vi "Refresh Targets.vi"(8 "Error In":errorcluster, 11 "Dependency Source Plugins":refnum<class "Dependency Source.lvclass">[](array[class])) -> (0 "Error Out":errorcluster, 1 "All Success?":bool, 2 "Success? Array":bool[](array[boolean]))   [LabVIEW 2019, in "Project.Dependencies Finder.lvlib"]
doc: "Refresh target lists for the given Dependency Source Plugins.\nProvider a Tracker to have a live view of the progress.\n\n2020-12-07: Henrik Dueholm Hansen"
uses:
  Project.Dependencies Finder.lvlib
  Dependency Source/Dependency Source.lvclass
panel:
  out "Target Refresh Progress":i32(slide) scale=0.0..100.0
  # "Refreshing targets. This may take a while.\nClose window to abort"
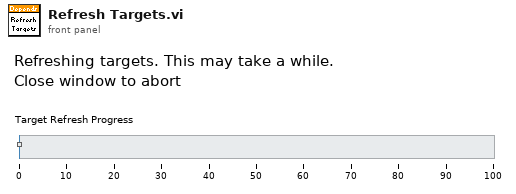
[diagram p1: front panel]
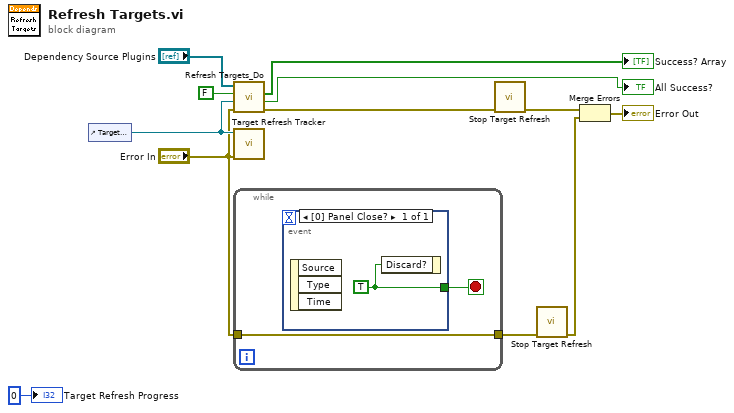
[diagram p0: block diagram]
diagram:
  n1 = control-ref of="Target Refresh Progress"() -> (w7:refnum<vi>)
  n2 = call "Refresh Targets_Do.vi"("Error In"="Error In", "Tracking Progress bar"=w7, "Allow UI?(T)"=FALSE ("Allow UI?"), "Dependency Source Plugins"="Dependency Source Plugins") -> ("Error Out"=w6:errorcluster, "All Success?"=→"All Success?":bool, "Success? Array"=→"Success? Array":bool[])  [unwired: 5 in]
  n3 = call "Target Refresh Tracker.vi"("Error In"="Error In", "Progress bar (auto closed)"=w7) -> ()  [unwired: 10 in]
  n4 = while {
    tunnel: "Error In" -> [w13]
    tunnel: [w13] -> w3
    stop <- w14 stop-if-true
    n5 = event shown="[0] Panel Close?" {
      selector: _ -> [_]
      dyn-events: _ -> [_]
      timeout: _ -> [_]
      tunnel: [w15] -> w14
      event Panel Close? {
        w15 = TRUE
        n6 = event-data() -> ()  [unwired: 1 in, 3 out]
        n7 = event-data("Discard?"=w15) -> ()  [unwired: 1 in, 1 out]
      }
    }
  }
  n8 = call "Stop Target Refresh.vi"("Error In"=w6) -> ("Error Out"=w5:errorcluster)  [unwired: 10 in]
  n9 = call "Stop Target Refresh.vi"("Error In"=w3) -> ("Error Out"=w1:errorcluster)  [unwired: 10 in]
  n10 = Merge Errors(w5, w1) -> (→"Error Out":errorcluster)
  "Target Refresh Progress" <- 0 ("Target Refresh Progress")
